vi "Array_Speed_test.vi"() -> ()   [LabVIEW 2010]
panel:
  in  "Array In 2":string[](array[string])
  in  "Boolean":bool
  out "x-y":u32
  out "Array 2":string[](array[string])
  in  "Array":i32[](array[numeric])
  in  "String":string
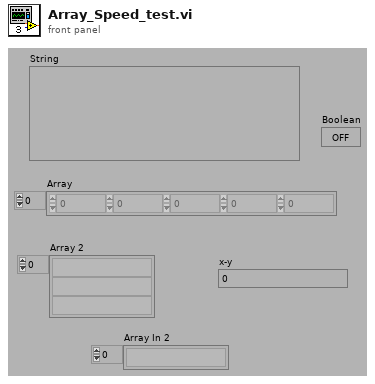
[diagram p1: front panel]
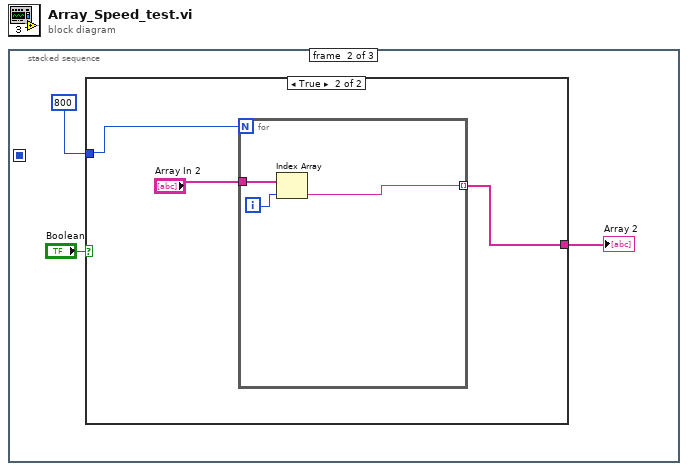
[diagram p0: block diagram]
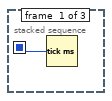
[diagram p2: hidden frame]
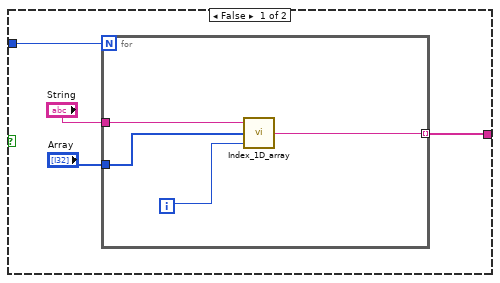
[diagram p3: hidden frame]
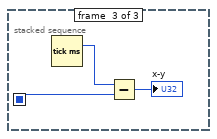
[diagram p4: hidden frame]
diagram:
  n1 = stacked-sequence {
    seq-local: [w1 _ _] -> [_ _ w21]
    frame #0 {
      n2 = Tick Count (ms)() -> (millisecond timer value=w1:u32)
    }
    frame #1 {
      n3 = case shown="True" "Boolean" {
        tunnel: [w5 w13] -> w4
        tunnel: 800 -> [w6 w15]
        frame False {
          n4 = for {
            N: w6 -> [_]
            tunnel: "String" -> [w12]
            tunnel: "Array" -> [w11]
            tunnel: [w9] -> w5 mode=indexing
            i -> [w10]
            n5 = call "Index_1D_array.vi"("Index"=w10, "Array"=w11, "String"=w12) -> ("String Element"=w9:string)
          }
        }
        frame True {
          n6 = for {
            N: w15 -> [_]
            tunnel: "Array In 2" -> [w18]
            tunnel: [w17] -> w13 mode=indexing
            i -> [w16]
            n7 = Index Array(array=w18, index=w16) -> (element=w17:string)
          }
        }
      }
      "Array 2" <- w4
    }
    frame #2 {
      n8 = Tick Count (ms)() -> (millisecond timer value=w20:u32)
      n9 = Subtract(x=w20, y=w21) -> (x-y=→"x-y":u32)
    }
  }
